vi "Chrg_Dschrg.vi"(0 "Data Task in":refnum<k21>, 1 "data task error in":errorcluster, 2 "#DAQ outputs (1-13)":i32, 4 "PS VISA in":refnum<visa-resource-name>, 5 "PS error in":errorcluster, 6 "DischargeCyclePath":path=path "C:/Users/ga11/Desktop/VI/results/3PtestCharge.lvm" caption="Filename", 8 "Charge/discharge":enum8{"Charge", "Discharge"}(ring), 9 "Charge/Discharge Voltage Setpoint":dbl format="%#.6g", 10 "CC or CCCV":enum16{"CC", "CCCV"}(ring), 11 "Current Setpoint":dbl format="%#.6g", 12 "Output Safety":T1, 13 "Current Cutoff":dbl) -> (14 "data task out":refnum<k21>, 15 "data task error out":errorcluster, 18 "PS VIS resource name out":refnum<visa-resource-name>, 19 "PS error out":errorcluster)   [LabVIEW 2020]
uses:
  Drivers-NHR-9200/NHR/Public/Data/Low Level/Fetch (Ave Voltage).vi
  Drivers-NHR-9200/NHR/NH Research Regenerative Test Series.lvlib
panel:
  out "Read Ave Current (A)":dbl
  out "Read Ave Voltage (V)":dbl
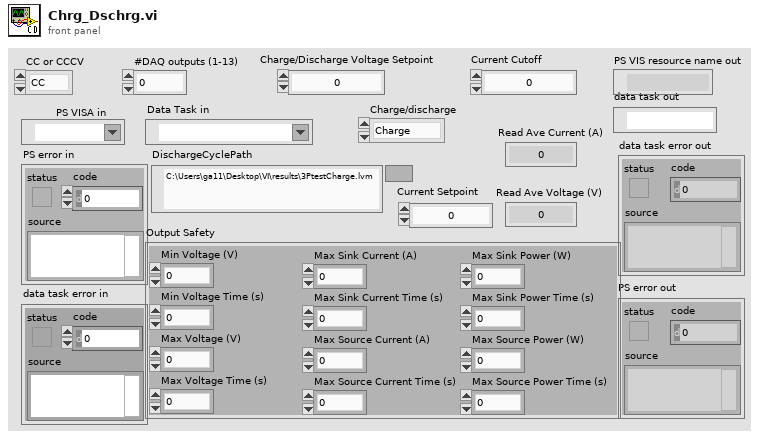
[diagram p1: front panel]
types:
  T1 = cluster{"Min Voltage (V)":dbl, "Min Voltage Time (s)":dbl, "Max Voltage (V)":dbl, "Max Voltage Time (s)":dbl, "Max Sink Current (A)":dbl, "Max Sink Current Time (s)":dbl, "Max Source Current (A)":dbl, "Max Source Current Time (s)":dbl, "Max Sink Power (W)":dbl, "Max Sink Power Time (s)":dbl, "Max Source Power (W)":dbl, "Max Source Power Time (s)":dbl}
  T2 = cluster{"Voltage Enabled":bool, "Current Enabled":bool, "Power Enabled":bool, "Resistance Enabled":bool}
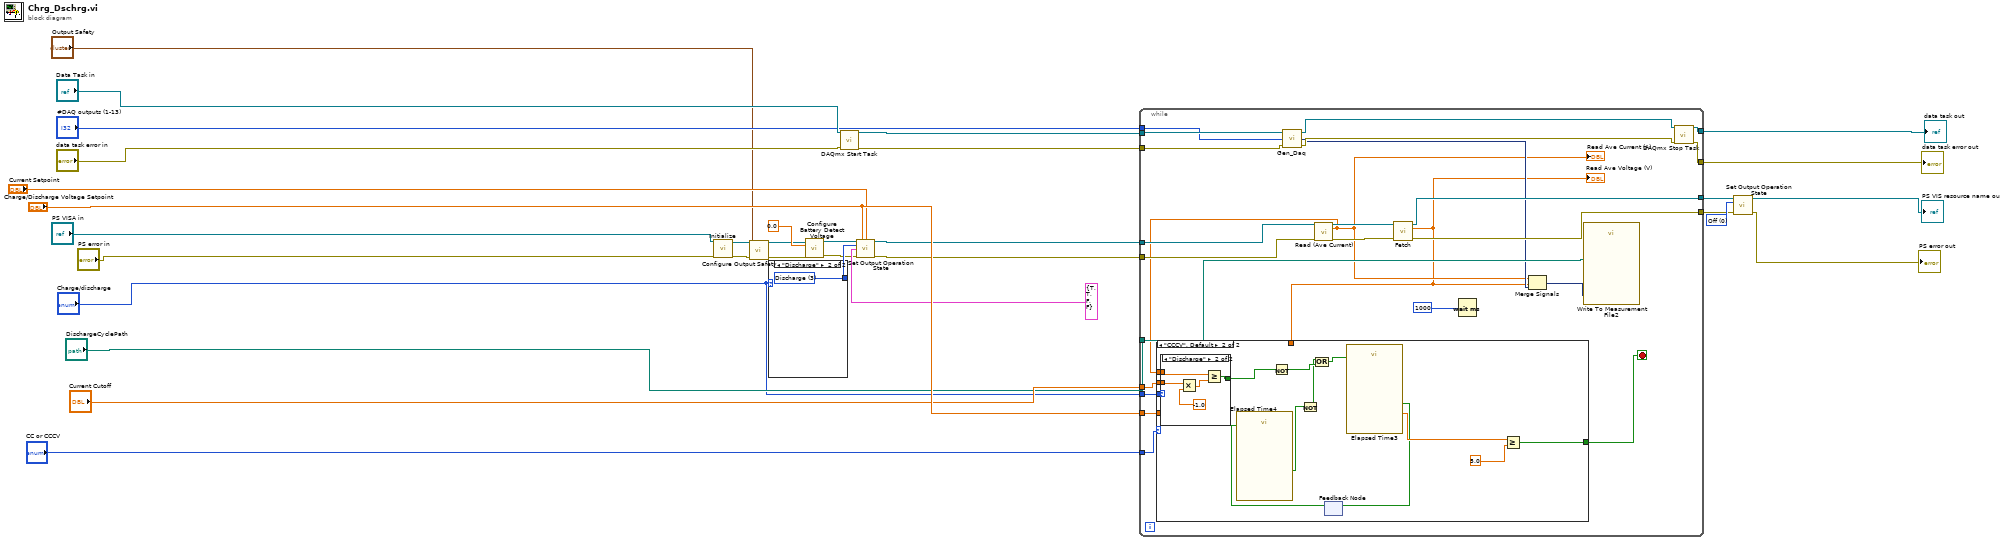
[diagram p0: block diagram]
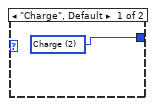
[diagram p2: hidden frame]
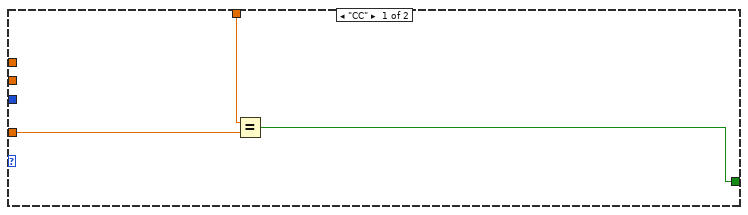
[diagram p3: hidden frame]
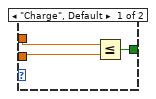
[diagram p4: hidden frame]
diagram:
  w13 = 0 items=["Off", "Standby", "Charge", "Discharge", "Battery"] ("Mode (0: Off)")
  n1 = call "Initialize.vi"("VISA resource name"="PS VISA in", "error in (no error)"="PS error in") -> ("VISA resource name out"=w4:refnum<visa-resource-name>, "error out"=w5:errorcluster)  [unwired: 12 in]
  n2 = call "Configure Output Safety.vi"("VISA resource name"=w4, "Output Safety"="Output Safety", "error in (no error)"=w5) -> ("VISA resource name out"=w7:refnum<visa-resource-name>, "error out"=w6:errorcluster)  [unwired: 11 in]
  n3 = case shown="\"Discharge\"" "Charge/discharge" {
    tunnel: [w33 w34] -> w16
    frame "Charge", Default {
      w33 = 2 items=["Off", "Standby", "Charge", "Discharge", "Battery"] ("Mode (0: Off)")
    }
    frame "Discharge" {
      w34 = 3 items=["Off", "Standby", "Charge", "Discharge", "Battery"] ("Mode (0: Off)")
    }
  }
  n4 = call "Configure Battery Detect Voltage.vi"("VISA resource name"=w7, "Battery Detect Voltage (0V)"=0.0, "error in (no error)"=w6) -> ("VISA resource name out"=w12:refnum<visa-resource-name>, "error out"=w11:errorcluster)  [unwired: 11 in]
  n5 = call <vilib>:"DAQmx Start Task.vi"("task/channels in"="Data Task in", "error in"="data task error in") -> ("task out"=w15:refnum<k21>, "error out"=w14:errorcluster)  [unwired: 12 in]
  n6 = call "Set Output Operation State.vi"("VISA resource name"=w12, "Voltage Setpoint (0 V)"="Charge/Discharge Voltage Setpoint", "Current Setpoint (0 A)"="Current Setpoint", "Mode (0: Off)"=w16, "Enable"=T2 {"Voltage Enabled"=TRUE, "Current Enabled"=TRUE, "Power Enabled"=FALSE, "Resistance Enabled"=FALSE}, "error in (no error)"=w11) -> ("VISA resource name out"=w19:refnum<visa-resource-name>, "error out"=w18:errorcluster)  [unwired: 8 in]
  n7 = while {
    tunnel: w19 -> [w56]
    tunnel: w18 -> [w55]
    tunnel: "Current Cutoff" -> [w40]
    tunnel: w14 -> [w45]
    tunnel: w15 -> [w46]
    tunnel: "DischargeCyclePath" -> [w51]
    tunnel: [w50] -> w26
    tunnel: [w49] -> w24
    tunnel: [w48] -> w9
    tunnel: [w47] -> w8
    tunnel: "#DAQ outputs (1-13)" -> [w44]
    tunnel: "CC or CCCV" -> [w38]
    tunnel: "Charge/Discharge Voltage Setpoint" -> [w36]
    tunnel: "Charge/discharge" -> [w35]
    stop <- w52 stop-if-true
    n8 = call "Gen_Daq.vi"("error in"=w45, "#DAQ outputs (1-13)"=w44, "task/channels in"=w46) -> ("error out"=w42:errorcluster, "DaQ_output"=w41:dynamicdata, "task out"=w43:refnum<k21>)
    n9 = call "Read (Ave Current).vi"("VISA resource name"=w56, "error in (no error)"=w55) -> ("VISA resource name out"=w57:refnum<visa-resource-name>, "Ave Current (A)"=w39:dbl, "error out"=w58:errorcluster)  [unwired: 11 in]
    "Read Ave Current (A)" <- w39
    n10 = call-poly "Fetch.vi"("VISA resource name"=w57, "error in (no error)"=w58) -> ("VISA resource name out"=w48:refnum<visa-resource-name>, "Ave Voltage (V)"=w37:dbl, "error out"=w47:errorcluster)  [unwired: 11 in]
    "Read Ave Voltage (V)" <- w37
    n11 = case shown="\"CCCV\", Default" w38 {
      tunnel: [w59 w68] -> w52
      tunnel: w40 -> [_ w65]
      tunnel: w39 -> [_ w64]
      tunnel: w37 -> [w61 _]
      tunnel: w36 -> [w60 _]
      tunnel: w35 -> [_ w62]
      frame "CC" {
        n12 = Equal?(x=w61, y=w60) -> (x = y?=w59:bool)
      }
      frame "CCCV", Default {
        n13 = case shown="\"Discharge\"" w62 {
          tunnel: w65 -> [w76 w81]
          tunnel: w64 -> [w77 w79]
          tunnel: [w75 w78] -> w63
          frame "Charge", Default {
            n14 = Less Or Equal?(x=w77, y=w76) -> (x <= y?=w75:bool)
          }
          frame "Discharge" {
            n15 = Multiply(x=w81, y=-1.0) -> (x*y=w80:dbl)
            n16 = Greater Or Equal?(x=w79, y=w80) -> (x >= y?=w78:bool)
          }
        }
        n17 = Not(x=w63) -> (.not. x?=w74:bool)
        n18 = feedback #1() -> (w66:bool)  [unwired: 1 in]
        n19 = call "Elapsed Time4"("Reset"=w66) -> ("Time has Elapsed"=w73:bool)  [unwired: 11 in, 7 out]
        n20 = Not(x=w73) -> (.not. x?=w72:bool)
        n21 = Or(x=w72, y=w74) -> (x .or. y?=w71:bool)
        n22 = call "Elapsed Time3"("Reset"=w71) -> ("Elapsed Time (s)"=w70:dbl, "Time has Elapsed"=w67:bool)  [unwired: 11 in, 6 out]
        n23 = feedback-in #1(w67) -> ()
        n24 = Greater Or Equal?(x=w70, y=5.0) -> (x >= y?=w68:bool)
      }
    }
    n25 = Wait (ms)(milliseconds to wait=1000) -> ()  [unwired: 1 out]
    n26 = Merge Signals "Merge Signals"(w39, w37, w41) -> (w54:dynamicdata)
    n27 = call "Write To Measurement File2"("Signals"=w54, "Filename"=w51) -> ()  [unwired: 15 in, 3 out]
    n28 = call <vilib>:"DAQmx Stop Task.vi"("task/channels in"=w43, "error in"=w42) -> ("task out"=w50:refnum<k21>, "error out"=w49:errorcluster)  [unwired: 12 in]
  }
  "data task out" <- w26
  "data task error out" <- w24
  n29 = call "Set Output Operation State.vi"("VISA resource name"=w9, "Mode (0: Off)"=w13, "error in (no error)"=w8) -> ("VISA resource name out"=→"PS VIS resource name out":refnum<visa-resource-name>, "error out"=→"PS error out":errorcluster)  [unwired: 11 in]
